vi "ULx-AIARG-UWKWT-Calibrate-Driver.vi"() -> ()   [LabVIEW 2017]
uses:
  <vilib>/Analysis/Matrix/Datatypes/RealMatrix.ctl
  <vilib>/Analysis/6fits.llb/Curve Fitting Criteria.ctl
  <vilib>/Analysis/baseanly.llb/Mean (DBL).vi
  <vilib>/ULx/Create Channel.llb/ULx Create Channel (AI-Voltage-Basic).vi
  <vilib>/ULx/Timing.llb/ULx Timing (Sample Clock).vi
  <vilib>/ULx/Read.llb/ULx Read (Analog Wfm 1Chan NSamp).vi
  <vilib>/Utility/file.llb/Write Delimited Spreadsheet (DBL).vi
  <vilib>/Analysis/Matrix/Numeric/Conversions/Array To Matrix - RA.vi
  <vilib>/Analysis/NI_AALBase.lvlib
  <vilib>/Analysis/Matrix/NI_Matrix.lvlib
  <vilib>/Analysis/NI_AALPro.lvlib
panel:
  out "CSV Array":dbl[][](array[numeric])
  in  "CSV Path":path
  in  "Rolling Moment Tab":T1(tab)
  out "Rolling Moment 1st Order Graph":T2(graph)
  out "Rolling Moment 1st Slope":dbl
  out "Rolling Moment 1st Intercept":dbl
  out "Rolling Moment 1st R-Squared":dbl
  out "Rolling Moment 2nd Order Graph":T2(graph)
  out "Rolling Moment 2nd Residue":dbl
  out "Rolling Moment 2nd Polynomial Coefficients":dbl[](array[numeric])
  out "Rolling Moment 3rd Order Graph":T2(graph)
  out "Rolling Moment 3rd Residue":dbl
  out "Rolling Moment 3rd Polynomial Coefficients":dbl[](array[numeric])
  in  "S.F. Tab":T3(tab)
  out "S.F. 1st Order Graph":cluster{"Weight":dbl[], "Voltage(S.F.)":dbl[]}[](graph)
  out "S.F. 1st Slope":dbl
  out "S.F. 1st Intercept":dbl
  out "S.F. 1st R-Squared":dbl
  out "S.F. 2nd Order Graph":cluster{"Weight":dbl[], "Voltage(S.F.)":dbl[]}[](graph)
  out "S.F. 2nd Polynomial Coefficients":dbl[](array[numeric])
  out "S.F. 2nd Residue":dbl
  out "S.F. 3rd Order Graph":cluster{"Weight":dbl[], "Voltage(S.F.)":dbl[]}[](graph)
  out "S.F. 3rd Polynomial Coefficients":dbl[](array[numeric])
  out "S.F. 3rd Residue":dbl
  in  "P.M. Tab":T4(tab)
  out "P.M. 1st Order Graph":cluster{"Weight":dbl[], "Voltage(P.M.)":dbl[]}[](graph)
  out "P.M. 1st Slope":dbl
  out "P.M. 1st Intercept":dbl
  out "P.M. 1st R-Squared":dbl
  out "P.M. 2nd Order Graph":cluster{"Weight":dbl[], "Voltage(P.M.)":dbl[]}[](graph)
  out "P.M. 2nd Polynomial Coefficients":dbl[](array[numeric])
  out "P.M. 2nd Residue":dbl
  out "P.M. 3rd Order Graph":cluster{"Weight":dbl[], "Voltage(P.M.)":dbl[]}[](graph)
  out "P.M. 3rd Polynomial Coefficients":dbl[](array[numeric])
  out "P.M. 3rd Residue":dbl
  in  "n Tab":enum32{"n Linear", "n 2nd Poly", "n 3rd Poly"}(tab)
  out "n 1st Order Graph":T5(graph)
  out "n 1st Slope":dbl
  out "n 1st Intercept":dbl
  out "n 1st R-Squared":dbl
  out "n 2nd Order Graph":T5(graph)
  out "n 2nd Residue":dbl
  out "n 2nd Polynomial Coefficients":dbl[](array[numeric])
  out "n 3rd Order Graph":T5(graph)
  out "n 3rd Polynomial Coefficients":dbl[](array[numeric])
  out "n 3rd Residue":dbl
  in  "Axial Tab":T6(tab)
  out "Axial 1st Order Graph":T7(graph)
  out "Axial 1st Slope":dbl
  out "Axial 1st Intercept":dbl
  out "Axial 1st R-Squared":dbl
  out "Axial 2nd Order Graph":T7(graph)
  out "Axial 2nd Residue":dbl
  out "Axial 2nd Polynomial Coefficients":dbl[](array[numeric])
  out "Axial 3rd Order Graph":T7(graph)
  out "Axial 3rd Polynomial Coefficients":dbl[](array[numeric])
  out "Axial 3rd Residue":dbl
  in  "Normal":T8(tab)
  out "Normal 1st Order Graph":T5(graph)
  out "Normal 1st Slope":dbl
  out "Normal 1st Intercept":dbl
  out "Normal 1st R-Squared":dbl
  out "Normal 2nd Order Graph":T5(graph)
  out "Normal 2nd Polynomial Coefficients":dbl[](array[numeric])
  out "Normal 2nd Residue":dbl
  out "Normal 3rd Order Graph":T5(graph)
  out "Normal 3rd Residue":dbl
  out "Normal 3rd Polynomial Coefficients":dbl[](array[numeric])
  out "Main Graph Intercept":dbl
  out "Main Graph R-Squared":dbl
  out "Main Graph Slope":dbl
  out "Main Graph":cluster{"Weight":dbl[], "Main Voltage":dbl[]}[](graph)
  out "Matrix Path Indicator":path
  in  "Report Path":path
  in  "Final Matrix":T9
  out "R.M. Sample Waveform":dbl[](graph)
  out "S.F. Sample Waveform":dbl[](graph)
  out "P.M. Sample Waveform":dbl[](graph)
  out "n Sample Waveform":dbl[](graph)
  out "Axial Force Sample Waveform":dbl[](graph)
  out "Normal Force Sample Waveform":dbl[](graph)
  out "Main Voltage":dbl[](array[numeric])
  out "Current Main Channel Calibration":string
  in  "Main Channel":string(combo)
  in  "Rolling Moment Physical Channel":refnum<k21>
  in  "S.F. Physical Channel":refnum<k21>
  in  "P.M. Physical Channel":refnum<k21>
  in  "n Physical Channel":refnum<k21>
  in  "Normal Force Physical Channel":refnum<k21>
  in  "minimum value":dbl=-5.0
  in  "maximum value":dbl=5.0
  in  "samples per channel":i32=100
  in  "sample mode":i32(ring) items=["FiniteSamples", "ContinuousSamples"]
  in  "rate":dbl=5000.0
  in  "Axial Force Physical Channel":refnum<k21>
  out "Voltage(R.M.)":dbl[](array[numeric])
  out "Voltage(S.F.)":dbl[](array[numeric])
  out "Voltage(P.M.)":dbl[](array[numeric])
  out "Voltage(n)":dbl[](array[numeric])
  out "Voltage(Normal)":dbl[](array[numeric])
  in  "Sample Button":bool
  in  "Add Weight":bool
  in  "Weight to be added":dbl
  out "Voltage(Axial)":dbl[](array[numeric])
  out "Weight":dbl[](array[numeric])
  in  "Clear Table":bool
  # "Channel and Sampling Selection"
  # "Interaction Plots\n\nPlots ALL SIX voltages,"
  # "Voltages from EACH Channel\nRecords data from all six channels for each sample cycle. Each number represents the mean of all values from one sample cycle recorded by one channel."
  # "Sample Waveform Graphs （For Debugging)\n\nPlots all the data points onto a waveform graph in one sample Cycle, to see the range of noises and determine any bias in data."
  # "Final Matrix\nThe final matrix that records the data from calibration and overwrites itself every time one calibration cycle is performed."
  # "Weight"
  # "Normal Force"
  # "Axial Force"
  # "n"
  # "P.M."
  # "S.F."
  # "Rolling Moment"
  # "f(x) ="
  # "*x +"
  # "f(x) ="
  # "*x +"
  # "f(x) ="
  # "*x +"
  # "f(x) ="
  # "*x +"
  # "f(x) ="
  # "*x +"
  # "f(x) ="
  # "*x +"
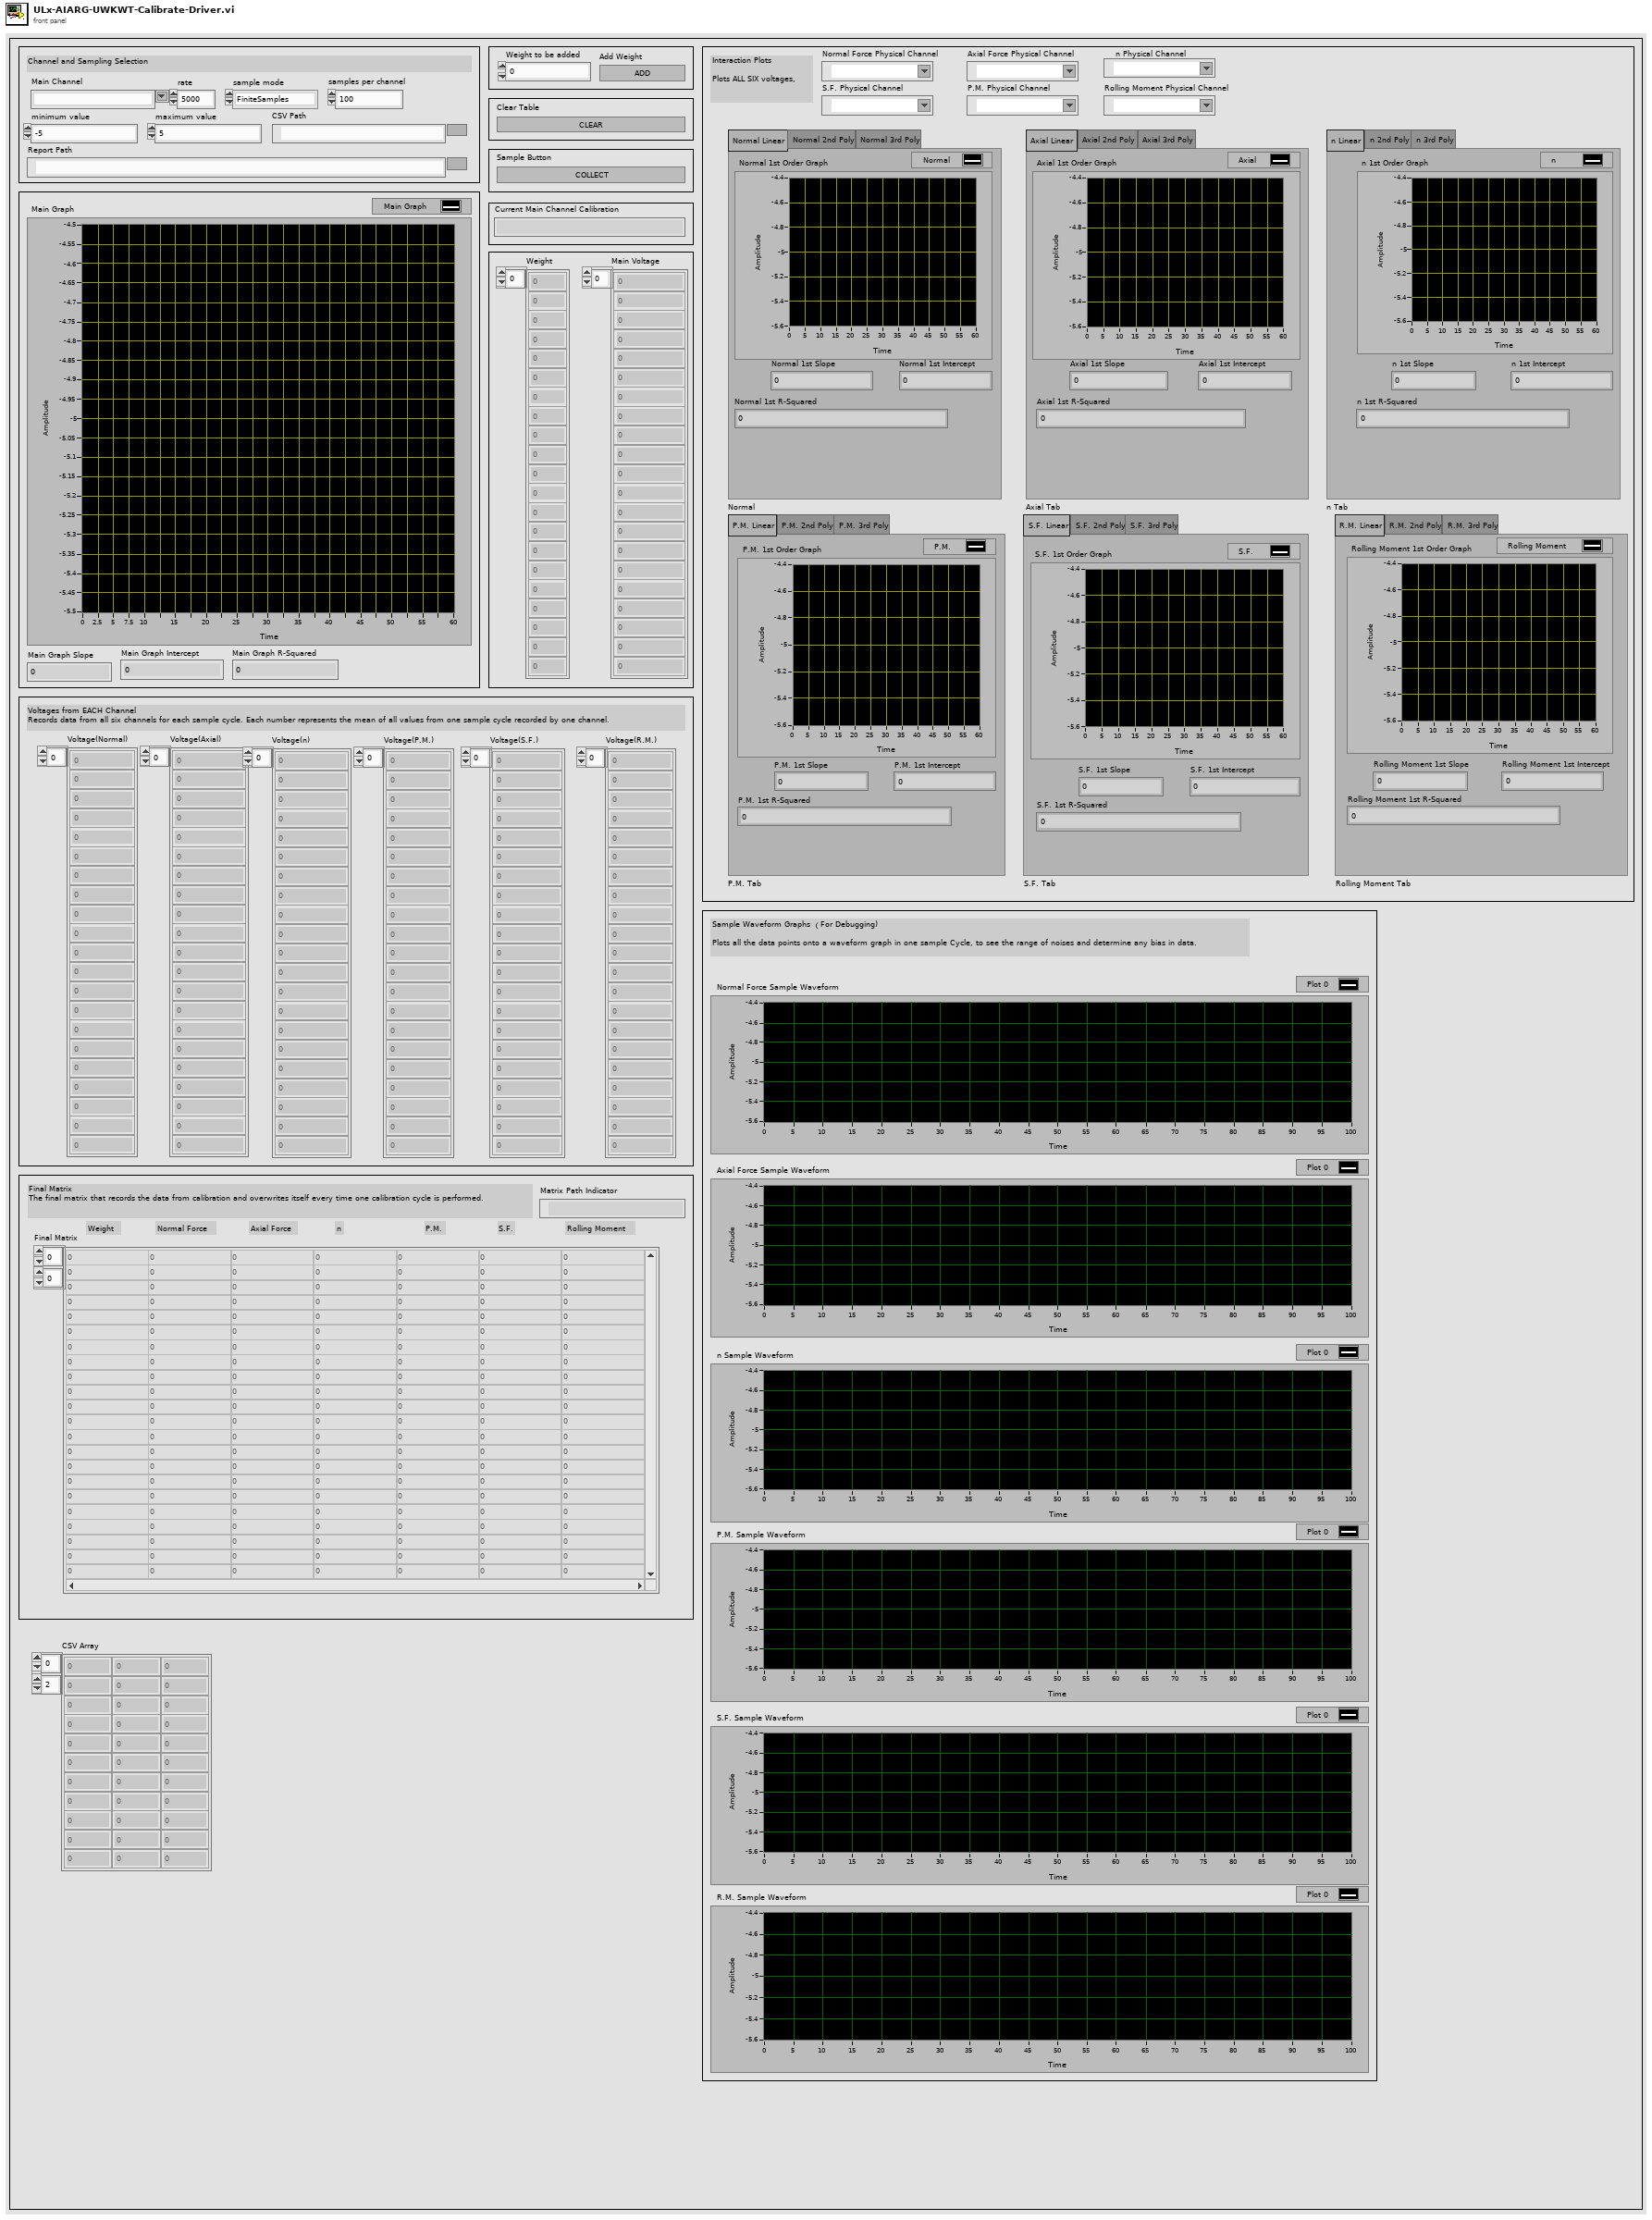
[diagram p1: front panel]
types:
  T1 = enum32{"R.M. Linear", "R.M. 2nd Poly", "R.M. 3rd Poly"}
  T2 = cluster{"Weight":dbl[], "Voltage(R.M.) ":dbl[]}[]
  T3 = enum32{"S.F. Linear", "S.F. 2nd Poly", "S.F. 3rd Poly"}
  T4 = enum32{"P.M. Linear", "P.M. 2nd Poly", "P.M. 3rd Poly"}
  T5 = cluster{"Weight":dbl[], "Best Linear Fit":dbl[]}[]
  T6 = enum32{"Axial Linear", "Axial 2nd Poly", "Axial 3rd Poly"}
  T7 = cluster{"Weight":dbl[], "Voltage(Axial)":dbl[]}[]
  T8 = enum32{"Normal Linear", "Normal 2nd Poly", "Normal 3rd Poly"}
  T9 = typedef "NI_Matrix.lvlib/RealMatrix.ctl" = dbl[][]
  T10 = typedef "NI_AALPro.lvlib/Curve Fitting Criteria.ctl" = u16
  T11 = cluster{"Weight":dbl[], "Best Polynomial Fit":dbl[]}
  T12 = cluster{"Weight":dbl[], "Best Polynomial Fit":dbl[]}[]
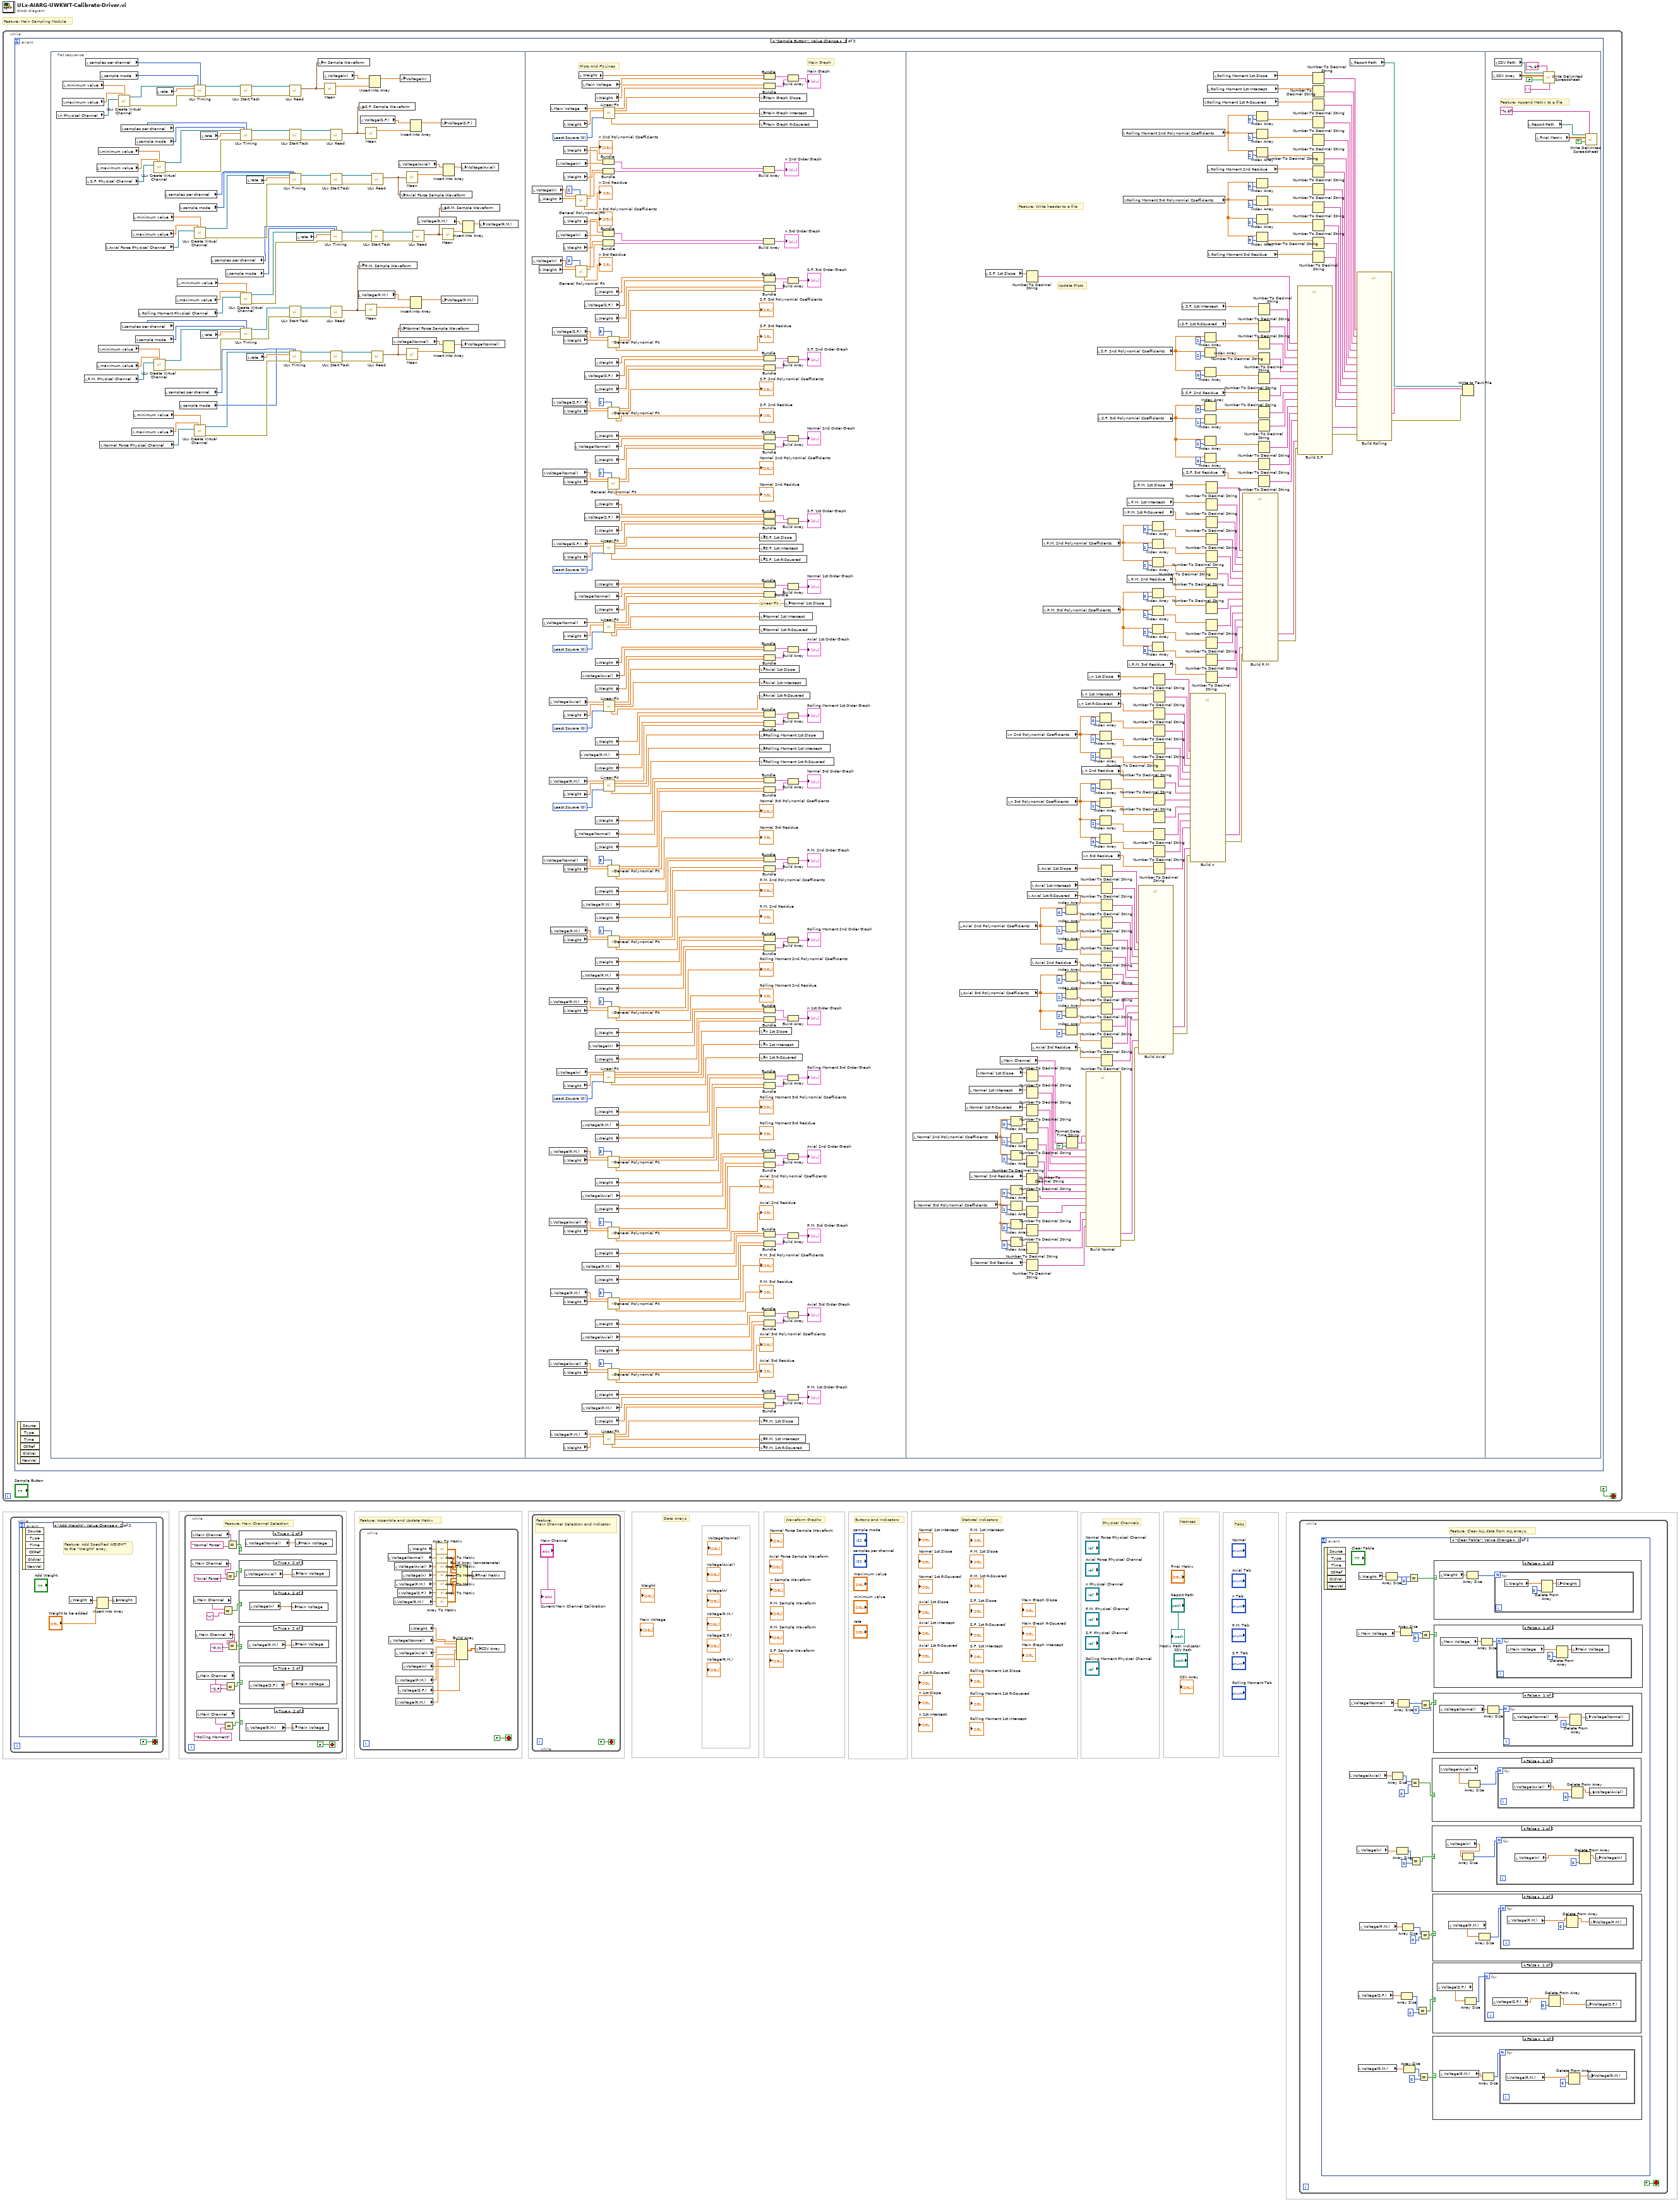
[diagram p0: block diagram]
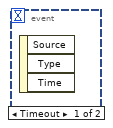
[diagram p8: hidden frame]
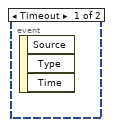
[diagram p17: hidden frame]
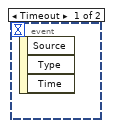
[diagram p18: hidden frame]
diagram:
  # "Tabs"
  # "Statistal Indicators"
  # "Matrices"
  # "Feature: Assemble and Update Matrix"
  # "Waveform Graphs"
  # "Physical Channels"
  # "Feature: Main Sampling Module"
  # "Data Arrays"
  # "Buttons and Indicators"
  n1 = while {
    stop <- FALSE stop-if-true
    n2 = event shown="[1] \"Sample Button\": Value Change" {
      selector: _ -> [_ _]
      dyn-events: _ -> [_ _]
      timeout: _ -> [_ _]
      event Timeout {
        n3 = event-data() -> ()  [unwired: 1 in, 3 out]
      }
      event "Sample Button": Value Change {
        n4 = event-data() -> ()  [unwired: 1 in, 6 out]
        n5 = flat-sequence {
          frame #0 {
            n6 = local read "n Physical Channel"() -> (w68:refnum<k21>)
            n7 = local read "maximum value"() -> (w64:dbl)
            n8 = local read "minimum value"() -> (w63:dbl)
            n9 = local read "P.M. Physical Channel"() -> (w53:refnum<k21>)
            n10 = local read "samples per channel"() -> (w66:i32)
            n11 = local read "S.F. Physical Channel"() -> (w28:refnum<k21>)
            n12 = local read "maximum value"() -> (w25:dbl)
            n13 = local read "maximum value"() -> (w52:dbl)
            n14 = local read "minimum value"() -> (w26:dbl)
            n15 = local read "minimum value"() -> (w51:dbl)
            n16 = local read "Normal Force Physical Channel"() -> (w83:refnum<k21>)
            n17 = local read "sample mode"() -> (w65:i32)
            n18 = local read "Axial Force Physical Channel"() -> (w84:refnum<k21>)
            n19 = call-poly <vilib>:"ULx Create Virtual Channel.vi"("maximum value"=w64, "minimum value"=w63, "physical channels"=w68) -> ("task out"=w54:refnum<k24>, "error out"=w55:errorcluster)  [unwired: 11 in]
            n20 = local read "samples per channel"() -> (w22:i32)
            n21 = local read "samples per channel"() -> (w43:i32)
            n22 = local read "maximum value"() -> (w88:dbl)
            n23 = local read "maximum value"() -> (w81:dbl)
            n24 = local read "minimum value"() -> (w95:dbl)
            n25 = local read "minimum value"() -> (w82:dbl)
            n26 = local read "sample mode"() -> (w21:i32)
            n27 = local read "sample mode"() -> (w42:i32)
            n28 = local read "Rolling Moment Physical Channel"() -> (w27:refnum<k21>)
            n29 = call-poly <vilib>:"ULx Create Virtual Channel.vi"("maximum value"=w25, "minimum value"=w26, "physical channels"=w28) -> ("task out"=w24:refnum<k24>, "error out"=w23:errorcluster)  [unwired: 11 in]
            n30 = call-poly <vilib>:"ULx Create Virtual Channel.vi"("maximum value"=w52, "minimum value"=w51, "physical channels"=w53) -> ("task out"=w50:refnum<k24>, "error out"=w41:errorcluster)  [unwired: 11 in]
            n31 = local read "rate"() -> (w67:dbl)
            n32 = local read "samples per channel"() -> (w85:i32)
            n33 = local read "samples per channel"() -> (w77:i32)
            n34 = local read "maximum value"() -> (w13:dbl)
            n35 = local read "minimum value"() -> (w14:dbl)
            n36 = local read "sample mode"() -> (w86:i32)
            n37 = local read "sample mode"() -> (w78:i32)
            n38 = call-poly <vilib>:"ULx Timing.vi"("task in"=w54, "sample mode"=w65, "samples per channel"=w66, "rate"=w67, "error in"=w55) -> ("task out"=w57:refnum<k24>, "error out"=w56:errorcluster)  [unwired: 9 in]
            n39 = call-poly <vilib>:"ULx Create Virtual Channel.vi"("maximum value"=w88, "minimum value"=w95, "physical channels"=w84) -> ("task out"=w89:refnum<k24>, "error out"=w94:errorcluster)  [unwired: 11 in]
            n40 = call-poly <vilib>:"ULx Create Virtual Channel.vi"("maximum value"=w81, "minimum value"=w82, "physical channels"=w83) -> ("task out"=w76:refnum<k24>, "error out"=w80:errorcluster)  [unwired: 11 in]
            n41 = local read "rate"() -> (w48:dbl)
            n42 = local read "rate"() -> (w49:dbl)
            n43 = local read "samples per channel"() -> (w16:i32)
            n44 = local read "sample mode"() -> (w15:i32)
            n45 = call <vilib>:"ULx Start Task.vi"("task in"=w57, "error in"=w56) -> ("task out"=w59:refnum<k24>, "error out"=w58:errorcluster)  [unwired: 12 in]
            n46 = call-poly <vilib>:"ULx Timing.vi"("task in"=w24, "sample mode"=w21, "samples per channel"=w22, "rate"=w48, "error in"=w23) -> ("task out"=w20:refnum<k24>, "error out"=w19:errorcluster)  [unwired: 9 in]
            n47 = call-poly <vilib>:"ULx Create Virtual Channel.vi"("maximum value"=w13, "minimum value"=w14, "physical channels"=w27) -> ("task out"=w12:refnum<k24>, "error out"=w11:errorcluster)  [unwired: 11 in]
            n48 = call-poly <vilib>:"ULx Timing.vi"("task in"=w50, "sample mode"=w42, "samples per channel"=w43, "rate"=w49, "error in"=w41) -> ("task out"=w40:refnum<k24>, "error out"=w39:errorcluster)  [unwired: 9 in]
            n49 = local read "rate"() -> (w87:dbl)
            n50 = local read "rate"() -> (w79:dbl)
            n51 = call-poly <vilib>:"ULx Read.vi"("task in"=w59, "error in"=w58) -> ("data"=w6:waveform(dbl))  [unwired: 11 in, 2 out]
            n52 = call <vilib>:"ULx Start Task.vi"("task in"=w20, "error in"=w19) -> ("task out"=w18:refnum<k24>, "error out"=w17:errorcluster)  [unwired: 12 in]
            n53 = call-poly <vilib>:"ULx Timing.vi"("task in"=w89, "sample mode"=w86, "samples per channel"=w85, "rate"=w87, "error in"=w94) -> ("task out"=w90:refnum<k24>, "error out"=w93:errorcluster)  [unwired: 9 in]
            n54 = call <vilib>:"ULx Start Task.vi"("task in"=w40, "error in"=w39) -> ("task out"=w38:refnum<k24>, "error out"=w37:errorcluster)  [unwired: 12 in]
            n55 = call-poly <vilib>:"ULx Timing.vi"("task in"=w76, "sample mode"=w78, "samples per channel"=w77, "rate"=w79, "error in"=w80) -> ("task out"=w75:refnum<k24>, "error out"=w74:errorcluster)  [unwired: 9 in]
            n56 = local read "rate"() -> (w47:dbl)
            n57 = local write "n Sample Waveform"(w6) -> ()
            n58 = local read "Voltage(n)"() -> (w62:dbl[])
            n59 = call-poly <vilib>:"Mean.vi"("X"=w6) -> ("mean"=w60:dbl)  [unwired: 1 out]
            n60 = call-poly <vilib>:"ULx Read.vi"("task in"=w18, "error in"=w17) -> ("data"=w3:waveform(dbl))  [unwired: 11 in, 2 out]
            n61 = call <vilib>:"ULx Start Task.vi"("task in"=w90, "error in"=w93) -> ("task out"=w91:refnum<k24>, "error out"=w92:errorcluster)  [unwired: 12 in]
            n62 = call-poly <vilib>:"ULx Timing.vi"("task in"=w12, "sample mode"=w15, "samples per channel"=w16, "rate"=w47, "error in"=w11) -> ("task out"=w10:refnum<k24>, "error out"=w9:errorcluster)  [unwired: 9 in]
            n63 = call-poly <vilib>:"ULx Read.vi"("task in"=w38, "error in"=w37) -> ("data"=w4:waveform(dbl))  [unwired: 11 in, 2 out]
            n64 = call <vilib>:"ULx Start Task.vi"("task in"=w75, "error in"=w74) -> ("task out"=w73:refnum<k24>, "error out"=w72:errorcluster)  [unwired: 12 in]
            n65 = local read "Voltage(P.M.)"() -> (w45:dbl[])
            n66 = local write "S.F. Sample Waveform"(w3) -> ()
            n67 = local write "P.M. Sample Waveform"(w4) -> ()
            n68 = local read "Voltage(S.F.)"() -> (w30:dbl[])
            n69 = call-poly <vilib>:"Mean.vi"("X"=w3) -> ("mean"=w31:dbl)  [unwired: 1 out]
            n70 = call-poly <vilib>:"Mean.vi"("X"=w4) -> ("mean"=w46:dbl)  [unwired: 1 out]
            n71 = Insert Into Array(array=w62, new element=w60) -> (w61:dbl[])  [unwired: 1 in]
            n72 = call-poly <vilib>:"ULx Read.vi"("task in"=w91, "error in"=w92) -> ("data"=w7:waveform(dbl))  [unwired: 11 in, 2 out]
            n73 = call <vilib>:"ULx Start Task.vi"("task in"=w10, "error in"=w9) -> ("task out"=w33:refnum<k24>, "error out"=w32:errorcluster)  [unwired: 12 in]
            n74 = call-poly <vilib>:"ULx Read.vi"("task in"=w73, "error in"=w72) -> ("data"=w8:waveform(dbl))  [unwired: 11 in, 2 out]
            n75 = local read "Voltage(Normal)"() -> (w70:dbl[])
            n76 = local read "Voltage(Axial)"() -> (w97:dbl[])
            n77 = local write "Voltage(n)"(w61) -> ()
            n78 = local write "Axial Force Sample Waveform"(w7) -> ()
            n79 = local write "Normal Force Sample Waveform"(w8) -> ()
            n80 = call-poly <vilib>:"Mean.vi"("X"=w7) -> ("mean"=w96:dbl)  [unwired: 1 out]
            n81 = call-poly <vilib>:"Mean.vi"("X"=w8) -> ("mean"=w71:dbl)  [unwired: 1 out]
            n82 = Insert Into Array(array=w30, new element=w31) -> (w29:dbl[])  [unwired: 1 in]
            n83 = Insert Into Array(array=w45, new element=w46) -> (w44:dbl[])  [unwired: 1 in]
            n84 = call-poly <vilib>:"ULx Read.vi"("task in"=w33, "error in"=w32) -> ("data"=w5:waveform(dbl))  [unwired: 11 in, 2 out]
            n85 = local read "Voltage(R.M.)"() -> (w35:dbl[])
            n86 = local write "Voltage(S.F.)"(w29) -> ()
            n87 = local write "R.M. Sample Waveform"(w5) -> ()
            n88 = local write "Voltage(P.M.)"(w44) -> ()
            n89 = call-poly <vilib>:"Mean.vi"("X"=w5) -> ("mean"=w34:dbl)  [unwired: 1 out]
            n90 = Insert Into Array(array=w97, new element=w96) -> (w98:dbl[])  [unwired: 1 in]
            n91 = Insert Into Array(array=w70, new element=w71) -> (w69:dbl[])  [unwired: 1 in]
            n92 = local write "Voltage(Axial)"(w98) -> ()
            n93 = local write "Voltage(Normal)"(w69) -> ()
            n94 = Insert Into Array(array=w35, new element=w34) -> (w36:dbl[])  [unwired: 1 in]
            n95 = local write "Voltage(R.M.)"(w36) -> ()
          }
          frame #1 {
            w223 = T10 0 items=["Least Square", "Least Absolute Residual", "Bisquare"] ("method")
            w247 = T10 0 items=["Least Square", "Least Absolute Residual", "Bisquare"] ("method")
            w275 = T10 0 items=["Least Square", "Least Absolute Residual", "Bisquare"] ("method")
            w286 = T10 0 items=["Least Square", "Least Absolute Residual", "Bisquare"] ("method")
            w297 = T10 0 items=["Least Square", "Least Absolute Residual", "Bisquare"] ("method")
            w312 = T10 0 items=["Least Square", "Least Absolute Residual", "Bisquare"] ("method")
            # "Main Graph"
            # "Linear Fit"
            # "Plots And Fit Lines"
            n96 = local read "Voltage(n)"() -> (w214:dbl[])
            n97 = local read "Voltage(n)"() -> (w139:dbl[])
            n98 = local read "Weight"() -> (w213:dbl[])
            n99 = local read "Weight"() -> (w138:dbl[])
            n100 = local read "Voltage(Normal)"() -> (w236:dbl[])
            n101 = local read "Voltage(Normal)"() -> (w301:dbl[])
            n102 = local read "Voltage(Normal)"() -> (w160:dbl[])
            n103 = local read "Voltage(Axial)"() -> (w288:dbl[])
            n104 = local read "Voltage(R.M.)"() -> (w246:dbl[])
            n105 = local read "Voltage(R.M.)"() -> (w179:dbl[])
            n106 = local read "Voltage(R.M.)"() -> (w106:dbl[])
            n107 = local read "Voltage(Axial)"() -> (w207:dbl[])
            n108 = local read "Voltage(Axial)"() -> (w150:dbl[])
            n109 = local read "Main Voltage"() -> (w316:dbl[])
            n110 = local read "Voltage(P.M.)"() -> (w186:dbl[])
            n111 = local read "Voltage(P.M.)"() -> (w127:dbl[])
            n112 = local read "Voltage(P.M.)"() -> (w266:dbl[])
            n113 = local read "Voltage(S.F.)"() -> (w113:dbl[])
            n114 = local read "Voltage(S.F.)"() -> (w201:dbl[])
            n115 = local read "Voltage(S.F.)"() -> (w259:dbl[])
            n116 = local read "Voltage(n)"() -> (w218:dbl[])
            n117 = local read "Voltage(n)"() -> (w144:dbl[])
            n118 = local read "Voltage(n)"() -> (w279:dbl[])
            n119 = local read "Weight"() -> (w317:dbl[])
            n120 = local read "Weight"() -> (w220:dbl[])
            n121 = local read "Weight"() -> (w215:dbl[])
            n122 = local read "Weight"() -> (w145:dbl[])
            n123 = local read "Weight"() -> (w143:dbl[])
            n124 = local read "Weight"() -> (w114:dbl[])
            n125 = local read "Weight"() -> (w200:dbl[])
            n126 = local read "Weight"() -> (w235:dbl[])
            n127 = local read "Weight"() -> (w258:dbl[])
            n128 = local read "Weight"() -> (w302:dbl[])
            n129 = local read "Weight"() -> (w287:dbl[])
            n130 = local read "Weight"() -> (w248:dbl[])
            n131 = local read "Weight"() -> (w159:dbl[])
            n132 = local read "Weight"() -> (w185:dbl[])
            n133 = local read "Weight"() -> (w178:dbl[])
            n134 = local read "Weight"() -> (w280:dbl[])
            n135 = local read "Weight"() -> (w107:dbl[])
            n136 = local read "Weight"() -> (w225:dbl[])
            n137 = local read "Weight"() -> (w126:dbl[])
            n138 = local read "Weight"() -> (w149:dbl[])
            n139 = local read "Weight"() -> (w265:dbl[])
            n140 = local read "Voltage(Normal)"() -> (w242:dbl[])
            n141 = local read "Voltage(Normal)"() -> (w330:dbl[])
            n142 = local read "Voltage(Normal)"() -> (w169:dbl[])
            n143 = call <vilib>:"General Polynomial Fit.vi"("Y"=w214, "polynomial order"=2, "X"=w213) -> ("Best Polynomial Fit"=w216:dbl[], "Polynomial Coefficients"=→"n 2nd Polynomial Coefficients":dbl[], "residue"=→"n 2nd Residue":dbl)  [unwired: 9 in, 1 out]
            n144 = call <vilib>:"General Polynomial Fit.vi"("Y"=w139, "polynomial order"=3, "X"=w138) -> ("Best Polynomial Fit"=w141:dbl[], "Polynomial Coefficients"=→"n 3rd Polynomial Coefficients":dbl[], "residue"=→"n 3rd Residue":dbl)  [unwired: 9 in, 1 out]
            n145 = local read "Weight"() -> (w311:dbl[])
            n146 = local read "Voltage(R.M.)"() -> (w320:dbl[])
            n147 = local read "Voltage(Axial)"() -> (w328:dbl[])
            n148 = local read "Voltage(R.M.)"() -> (w181:dbl[])
            n149 = local read "Voltage(R.M.)"() -> (w109:dbl[])
            n150 = local read "Voltage(Axial)"() -> (w208:dbl[])
            n151 = local read "Voltage(Axial)"() -> (w157:dbl[])
            n152 = local read "Main Voltage"() -> (w332:dbl[])
            n153 = local read "Voltage(P.M.)"() -> (w190:dbl[])
            n154 = local read "Voltage(P.M.)"() -> (w133:dbl[])
            n155 = local read "Voltage(P.M.)"() -> (w324:dbl[])
            n156 = local read "Voltage(S.F.)"() -> (w121:dbl[])
            n157 = local read "Voltage(S.F.)"() -> (w205:dbl[])
            n158 = local read "Voltage(S.F.)"() -> (w322:dbl[])
            n159 = local read "Voltage(n)"() -> (w326:dbl[])
            n160 = local read "Weight"() -> (w309:dbl[])
            n161 = local read "Weight"() -> (w122:dbl[])
            n162 = local read "Weight"() -> (w119:dbl[])
            n163 = local read "Weight"() -> (w206:dbl[])
            n164 = local read "Weight"() -> (w203:dbl[])
            n165 = local read "Weight"() -> (w243:dbl[])
            n166 = local read "Weight"() -> (w239:dbl[])
            n167 = local read "Weight"() -> (w323:dbl[])
            n168 = local read "Weight"() -> (w260:dbl[])
            n169 = local read "Weight"() -> (w331:dbl[])
            n170 = local read "Weight"() -> (w307:dbl[])
            n171 = local read "Weight"() -> (w329:dbl[])
            n172 = local read "Weight"() -> (w293:dbl[])
            n173 = local read "Weight"() -> (w321:dbl[])
            n174 = local read "Weight"() -> (w245:dbl[])
            n175 = local read "Weight"() -> (w170:dbl[])
            n176 = local read "Weight"() -> (w168:dbl[])
            n177 = local read "Weight"() -> (w191:dbl[])
            n178 = local read "Weight"() -> (w189:dbl[])
            n179 = local read "Weight"() -> (w182:dbl[])
            n180 = local read "Weight"() -> (w177:dbl[])
            n181 = local read "Weight"() -> (w327:dbl[])
            n182 = local read "Weight"() -> (w285:dbl[])
            n183 = local read "Weight"() -> (w110:dbl[])
            n184 = local read "Weight"() -> (w108:dbl[])
            n185 = local read "Weight"() -> (w231:dbl[])
            n186 = local read "Weight"() -> (w230:dbl[])
            n187 = local read "Weight"() -> (w134:dbl[])
            n188 = local read "Weight"() -> (w131:dbl[])
            n189 = local read "Weight"() -> (w158:dbl[])
            n190 = local read "Weight"() -> (w156:dbl[])
            n191 = local read "Weight"() -> (w325:dbl[])
            n192 = local read "Weight"() -> (w271:dbl[])
            n193 = Bundle("Weight"=w220, "Voltage(n)"=w218) -> (w219:cluster{"Weight":dbl[], "Voltage(n)":dbl[]})  [unwired: 1 in]
            n194 = Bundle("Weight"=w215, "Best Polynomial Fit"=w216) -> (w217:T11)  [unwired: 1 in]
            n195 = Bundle("Weight"=w145, "Voltage(n)"=w144) -> (w146:cluster{"Weight":dbl[], "Voltage(n)":dbl[]})  [unwired: 1 in]
            n196 = Bundle("Weight"=w143, "Best Polynomial Fit"=w141) -> (w142:T11)  [unwired: 1 in]
            n197 = call <vilib>:"Linear Fit.vi"("Y"=w316, "X"=w317, "method"=w312) -> ("Best Linear Fit"=w308:dbl[], "slope"=w315:dbl, "intercept"=w314:dbl, "residue"=w313:dbl)  [unwired: 8 in, 1 out]
            n198 = call <vilib>:"Linear Fit.vi"("Y"=w259, "X"=w258, "method"=w247) -> ("Best Linear Fit"=w261:dbl[], "slope"=w257:dbl, "intercept"=w256:dbl, "residue"=w255:dbl)  [unwired: 8 in, 1 out]
            n199 = call <vilib>:"Linear Fit.vi"("Y"=w301, "X"=w302, "method"=w297) -> ("Best Linear Fit"=w304:dbl[], "slope"=w303:dbl, "intercept"=w305:dbl, "residue"=w306:dbl)  [unwired: 8 in, 1 out]
            n200 = call <vilib>:"Linear Fit.vi"("Y"=w288, "X"=w287, "method"=w286) -> ("Best Linear Fit"=w292:dbl[], "slope"=w291:dbl, "intercept"=w290:dbl, "residue"=w289:dbl)  [unwired: 8 in, 1 out]
            n201 = call <vilib>:"Linear Fit.vi"("Y"=w246, "X"=w248, "method"=w223) -> ("Best Linear Fit"=w252:dbl[], "slope"=w251:dbl, "intercept"=w250:dbl, "residue"=w249:dbl)  [unwired: 8 in, 1 out]
            n202 = call <vilib>:"Linear Fit.vi"("Y"=w279, "X"=w280, "method"=w275) -> ("Best Linear Fit"=w284:dbl[], "slope"=w283:dbl, "intercept"=w282:dbl, "residue"=w281:dbl)  [unwired: 8 in, 1 out]
            n203 = call <vilib>:"Linear Fit.vi"("Y"=w266, "X"=w265) -> ("Best Linear Fit"=w272:dbl[], "slope"=w269:dbl, "intercept"=w268:dbl, "residue"=w267:dbl)  [unwired: 9 in, 1 out]
            n204 = call <vilib>:"General Polynomial Fit.vi"("Y"=w113, "polynomial order"=3, "X"=w114) -> ("Best Polynomial Fit"=w118:dbl[], "Polynomial Coefficients"=→"S.F. 3rd Polynomial Coefficients":dbl[], "residue"=→"S.F. 3rd Residue":dbl)  [unwired: 9 in, 1 out]
            n205 = call <vilib>:"General Polynomial Fit.vi"("Y"=w201, "polynomial order"=2, "X"=w200) -> ("Best Polynomial Fit"=w202:dbl[], "Polynomial Coefficients"=→"S.F. 2nd Polynomial Coefficients":dbl[], "residue"=→"S.F. 2nd Residue":dbl)  [unwired: 9 in, 1 out]
            n206 = call <vilib>:"General Polynomial Fit.vi"("Y"=w236, "polynomial order"=2, "X"=w235) -> ("Best Polynomial Fit"=w238:dbl[], "Polynomial Coefficients"=→"Normal 2nd Polynomial Coefficients":dbl[], "residue"=→"Normal 2nd Residue":dbl)  [unwired: 9 in, 1 out]
            n207 = call <vilib>:"General Polynomial Fit.vi"("Y"=w160, "polynomial order"=3, "X"=w159) -> ("Best Polynomial Fit"=w167:dbl[], "Polynomial Coefficients"=→"Normal 3rd Polynomial Coefficients":dbl[], "residue"=→"Normal 3rd Residue":dbl)  [unwired: 9 in, 1 out]
            n208 = call <vilib>:"General Polynomial Fit.vi"("Y"=w186, "polynomial order"=2, "X"=w185) -> ("Best Polynomial Fit"=w188:dbl[], "Polynomial Coefficients"=→"P.M. 2nd Polynomial Coefficients":dbl[], "residue"=→"P.M. 2nd Residue":dbl)  [unwired: 9 in, 1 out]
            n209 = call <vilib>:"General Polynomial Fit.vi"("Y"=w179, "polynomial order"=2, "X"=w178) -> ("Best Polynomial Fit"=w180:dbl[], "Polynomial Coefficients"=→"Rolling Moment 2nd Polynomial Coefficients":dbl[], "residue"=→"Rolling Moment 2nd Residue":dbl)  [unwired: 9 in, 1 out]
            n210 = call <vilib>:"General Polynomial Fit.vi"("Y"=w106, "polynomial order"=3, "X"=w107) -> ("Best Polynomial Fit"=w104:dbl[], "Polynomial Coefficients"=→"Rolling Moment 3rd Polynomial Coefficients":dbl[], "residue"=→"Rolling Moment 3rd Residue":dbl)  [unwired: 9 in, 1 out]
            n211 = call <vilib>:"General Polynomial Fit.vi"("Y"=w207, "polynomial order"=2, "X"=w225) -> ("Best Polynomial Fit"=w227:dbl[], "Polynomial Coefficients"=→"Axial 2nd Polynomial Coefficients":dbl[], "residue"=→"Axial 2nd Residue":dbl)  [unwired: 9 in, 1 out]
            n212 = call <vilib>:"General Polynomial Fit.vi"("Y"=w127, "polynomial order"=3, "X"=w126) -> ("Best Polynomial Fit"=w132:dbl[], "Polynomial Coefficients"=→"P.M. 3rd Polynomial Coefficients":dbl[], "residue"=→"P.M. 3rd Residue":dbl)  [unwired: 9 in, 1 out]
            n213 = call <vilib>:"General Polynomial Fit.vi"("Y"=w150, "polynomial order"=3, "X"=w149) -> ("Best Polynomial Fit"=w154:dbl[], "Polynomial Coefficients"=→"Axial 3rd Polynomial Coefficients":dbl[], "residue"=→"Axial 3rd Residue":dbl)  [unwired: 9 in, 1 out]
            n214 = local write "Main Graph Slope"(w315) -> ()
            n215 = local write "Main Graph Intercept"(w314) -> ()
            n216 = local write "Main Graph R-Squared"(w313) -> ()
            n217 = local write "S.F. 1st Slope"(w257) -> ()
            n218 = local write "S.F. 1st Intercept"(w256) -> ()
            n219 = local write "S.F. 1st R-Squared"(w255) -> ()
            n220 = local write "Normal 1st Intercept"(w305) -> ()
            n221 = local write "Normal 1st R-Squared"(w306) -> ()
            n222 = local write "Axial 1st Slope"(w291) -> ()
            n223 = local write "Axial 1st Intercept"(w290) -> ()
            n224 = local write "Axial 1st R-Squared"(w289) -> ()
            n225 = local write "Rolling Moment 1st Slope"(w251) -> ()
            n226 = local write "Rolling Moment 1st Intercept"(w250) -> ()
            n227 = local write "Rolling Moment 1st R-Squared"(w249) -> ()
            n228 = local write "n 1st Slope"(w283) -> ()
            n229 = local write "n 1st Intercept"(w282) -> ()
            n230 = local write "n 1st R-Squared"(w281) -> ()
            n231 = local write "P.M. 1st Slope"(w269) -> ()
            n232 = local write "P.M. 1st Intercept"(w268) -> ()
            n233 = local write "P.M. 1st R-Squared"(w267) -> ()
            n234 = Build Array(w219, w217) -> (→"n 2nd Order Graph":T12)
            n235 = Build Array(w146, w142) -> (→"n 3rd Order Graph":T12)
            n236 = Bundle("Weight"=w311, "Main Voltage"=w332) -> (w318:cluster{"Weight":dbl[], "Main Voltage":dbl[]})  [unwired: 1 in]
            n237 = Bundle("Weight"=w309, "Best Linear Fit"=w308) -> (w310:cluster{"Weight":dbl[], "Best Linear Fit":dbl[]})  [unwired: 1 in]
            n238 = Bundle("Weight"=w122, "Voltage(S.F.)"=w121) -> (w120:cluster{"Weight":dbl[], "Voltage(S.F.)":dbl[]})  [unwired: 1 in]
            n239 = Bundle("Weight"=w119, "Best Polynomial Fit"=w118) -> (w111:T11)  [unwired: 1 in]
            n240 = Bundle("Weight"=w206, "Voltage(S.F.)"=w205) -> (w204:cluster{"Weight":dbl[], "Voltage(S.F.)":dbl[]})  [unwired: 1 in]
            n241 = Bundle("Weight"=w203, "Best Polynomial Fit"=w202) -> (w199:T11)  [unwired: 1 in]
            n242 = Bundle("Weight"=w243, "Voltage(Normal)"=w242) -> (w241:cluster{"Weight":dbl[], "Voltage(Normal)":dbl[]})  [unwired: 1 in]
            n243 = Bundle("Weight"=w239, "Best Polynomial Fit"=w238) -> (w237:T11)  [unwired: 1 in]
            n244 = Bundle("Weight"=w323, "Voltage(S.F.)"=w322) -> (w263:cluster{"Weight":dbl[], "Voltage(S.F.)":dbl[]})  [unwired: 1 in]
            n245 = Bundle("Weight"=w260, "Best Linear Fit"=w261) -> (w262:cluster{"Weight":dbl[], "Best Linear Fit":dbl[]})  [unwired: 1 in]
            n246 = Bundle("Weight"=w331, "Voltage(Normal)"=w330) -> (w300:cluster{"Weight":dbl[], "Voltage(Normal)":dbl[]})  [unwired: 1 in]
            n247 = Bundle("Weight"=w307, "Best Linear Fit"=w304) -> (w299:cluster{"Weight":dbl[], "Best Linear Fit":dbl[]})  [unwired: 1 in]
            n248 = Bundle("Weight"=w329, "Voltage(Axial)"=w328) -> (w295:cluster{"Weight":dbl[], "Voltage(Axial)":dbl[]})  [unwired: 1 in]
            n249 = Bundle("Weight"=w293, "Best Linear Fit"=w292) -> (w294:cluster{"Weight":dbl[], "Best Linear Fit":dbl[]})  [unwired: 1 in]
            n250 = Bundle("Weight"=w321, "Voltage(R.M.)"=w320) -> (w253:cluster{"Weight":dbl[], "Voltage(R.M.) ":dbl[]})  [unwired: 1 in]
            n251 = Bundle("Weight"=w245, "Best Linear Fit"=w252) -> (w244:cluster{"Weight":dbl[], "Best Linear Fit":dbl[]})  [unwired: 1 in]
            n252 = Bundle("Weight"=w170, "Voltage(Normal)"=w169) -> (w163:cluster{"Weight":dbl[], "Voltage(Normal)":dbl[]})  [unwired: 1 in]
            n253 = Bundle("Weight"=w168, "Best Polynomial Fit"=w167) -> (w161:T11)  [unwired: 1 in]
            n254 = Bundle("Weight"=w191, "Voltage(P.M.)"=w190) -> (w193:cluster{"Weight":dbl[], "Voltage(P.M.)":dbl[]})  [unwired: 1 in]
            n255 = Bundle("Weight"=w189, "Best Polynomial Fit"=w188) -> (w192:T11)  [unwired: 1 in]
            n256 = Bundle("Weight"=w182, "Voltage(R.M.)"=w181) -> (w172:cluster{"Weight":dbl[], "Voltage(R.M.) ":dbl[]})  [unwired: 1 in]
            n257 = Bundle("Weight"=w177, "Best Polynomial Fit"=w180) -> (w173:T11)  [unwired: 1 in]
            n258 = Bundle("Weight"=w327, "Voltage(n)"=w326) -> (w278:cluster{"Weight":dbl[], "Voltage(n)":dbl[]})  [unwired: 1 in]
            n259 = Bundle("Weight"=w285, "Best Linear Fit"=w284) -> (w277:cluster{"Weight":dbl[], "Best Linear Fit":dbl[]})  [unwired: 1 in]
            n260 = Bundle("Weight"=w110, "Voltage(R.M.)"=w109) -> (w103:cluster{"Weight":dbl[], "Voltage(R.M.) ":dbl[]})  [unwired: 1 in]
            n261 = Bundle("Weight"=w108, "Best Polynomial Fit"=w104) -> (w102:T11)  [unwired: 1 in]
            n262 = Bundle("Weight"=w231, "Voltage(Axial)"=w208) -> (w229:cluster{"Weight":dbl[], "Voltage(Axial)":dbl[]})  [unwired: 1 in]
            n263 = Bundle("Weight"=w230, "Best Polynomial Fit"=w227) -> (w228:T11)  [unwired: 1 in]
            n264 = Bundle("Weight"=w134, "Voltage(P.M.)"=w133) -> (w130:cluster{"Weight":dbl[], "Voltage(P.M.)":dbl[]})  [unwired: 1 in]
            n265 = Bundle("Weight"=w131, "Best Polynomial Fit"=w132) -> (w129:T11)  [unwired: 1 in]
            n266 = Bundle("Weight"=w158, "Voltage(Axial)"=w157) -> (w153:cluster{"Weight":dbl[], "Voltage(Axial)":dbl[]})  [unwired: 1 in]
            n267 = Bundle("Weight"=w156, "Best Polynomial Fit"=w154) -> (w152:T11)  [unwired: 1 in]
            n268 = Bundle("Weight"=w325, "Voltage(P.M.)"=w324) -> (w273:cluster{"Weight":dbl[], "Voltage(P.M.)":dbl[]})  [unwired: 1 in]
            n269 = Bundle("Weight"=w271, "Best Linear Fit"=w272) -> (w270:cluster{"Weight":dbl[], "Best Linear Fit":dbl[]})  [unwired: 1 in]
            n270 = local write "Normal 1st Slope"(w303) -> ()
            n271 = Build Array(w318, w310) -> (→"Main Graph":T5)
            n272 = Build Array(w120, w111) -> (→"S.F. 3rd Order Graph":T12)
            n273 = Build Array(w204, w199) -> (→"S.F. 2nd Order Graph":T12)
            n274 = Build Array(w241, w237) -> (→"Normal 2nd Order Graph":T12)
            n275 = Build Array(w263, w262) -> (→"S.F. 1st Order Graph":T5)
            n276 = Build Array(w300, w299) -> (→"Normal 1st Order Graph":T5)
            n277 = Build Array(w295, w294) -> (→"Axial 1st Order Graph":T5)
            n278 = Build Array(w253, w244) -> (→"Rolling Moment 1st Order Graph":T5)
            n279 = Build Array(w163, w161) -> (→"Normal 3rd Order Graph":T12)
            n280 = Build Array(w193, w192) -> (→"P.M. 2nd Order Graph":T12)
            n281 = Build Array(w172, w173) -> (→"Rolling Moment 2nd Order Graph":T12)
            n282 = Build Array(w278, w277) -> (→"n 1st Order Graph":T5)
            n283 = Build Array(w103, w102) -> (→"Rolling Moment 3rd Order Graph":T12)
            n284 = Build Array(w229, w228) -> (→"Axial 2nd Order Graph":T12)
            n285 = Build Array(w130, w129) -> (→"P.M. 3rd Order Graph":T12)
            n286 = Build Array(w153, w152) -> (→"Axial 3rd Order Graph":T12)
            n287 = Build Array(w273, w270) -> (→"P.M. 1st Order Graph":T5)
          }
          frame #2 {
            # "Feature: Write header to a file"
            # "Update Plots"
            n288 = local read "Normal 2nd Polynomial Coefficients"() -> (w531:dbl[])
            n289 = local read "Normal 3rd Polynomial Coefficients"() -> (w523:dbl[])
            n290 = local read "Axial 2nd Polynomial Coefficients"() -> (w499:dbl[])
            n291 = local read "Axial 3rd Polynomial Coefficients"() -> (w489:dbl[])
            n292 = local read "Normal 1st R-Squared"() -> (w539:dbl)
            n293 = local read "Normal 1st Intercept"() -> (w541:dbl)
            n294 = local read "Normal 2nd Residue"() -> (w537:dbl)
            n295 = local read "Normal 3rd Residue"() -> (w534:dbl)
            n296 = local read "Normal 1st Slope"() -> (w543:dbl)
            n297 = local read "S.F. 1st Slope"() -> (w403:dbl)
            n298 = local read "Main Channel"() -> (w545:string)
            n299 = local read "n 2nd Polynomial Coefficients"() -> (w457:dbl[])
            n300 = local read "n 3rd Polynomial Coefficients"() -> (w450:dbl[])
            n301 = Index Array(array=w531, index=0) -> (element=w533:dbl)
            n302 = Index Array(array=w531, index=1) -> (element=w528:dbl)
            n303 = Index Array(array=w531, index=2) -> (element=w527:dbl)
            n304 = Index Array(array=w523, index=0) -> (element=w518:dbl)
            n305 = Index Array(array=w523, index=1) -> (element=w517:dbl)
            n306 = Index Array(array=w523, index=2) -> (element=w516:dbl)
            n307 = Index Array(array=w523, index=3) -> (element=w515:dbl)
            n308 = Number To Decimal String(number=w403) -> (decimal integer string=w400:string)  [unwired: 1 in]
            n309 = Number To Decimal String(number=w543) -> (decimal integer string=w542:string)  [unwired: 1 in]
            n310 = Number To Decimal String(number=w541) -> (decimal integer string=w540:string)  [unwired: 1 in]
            n311 = Number To Decimal String(number=w539) -> (decimal integer string=w538:string)  [unwired: 1 in]
            n312 = Number To Decimal String(number=w533) -> (decimal integer string=w526:string)  [unwired: 1 in]
            n313 = Number To Decimal String(number=w528) -> (decimal integer string=w525:string)  [unwired: 1 in]
            n314 = Number To Decimal String(number=w527) -> (decimal integer string=w524:string)  [unwired: 1 in]
            n315 = Number To Decimal String(number=w537) -> (decimal integer string=w536:string)  [unwired: 1 in]
            n316 = Number To Decimal String(number=w518) -> (decimal integer string=w514:string)  [unwired: 1 in]
            n317 = Number To Decimal String(number=w517) -> (decimal integer string=w513:string)  [unwired: 1 in]
            n318 = Number To Decimal String(number=w516) -> (decimal integer string=w512:string)  [unwired: 1 in]
            n319 = Number To Decimal String(number=w515) -> (decimal integer string=w511:string)  [unwired: 1 in]
            n320 = Number To Decimal String(number=w534) -> (decimal integer string=w535:string)  [unwired: 1 in]
            n321 = local read "Axial 1st R-Squared"() -> (w505:dbl)
            n322 = local read "Axial 1st Intercept"() -> (w507:dbl)
            n323 = local read "Axial 2nd Residue"() -> (w503:dbl)
            n324 = local read "Axial 3rd Residue"() -> (w501:dbl)
            n325 = local read "Axial 1st Slope"() -> (w509:dbl)
            n326 = local read "P.M. 2nd Polynomial Coefficients"() -> (w428:dbl[])
            n327 = local read "P.M. 3rd Polynomial Coefficients"() -> (w427:dbl[])
            n328 = Index Array(array=w499, index=0) -> (element=w495:dbl)
            n329 = Index Array(array=w499, index=1) -> (element=w494:dbl)
            n330 = Index Array(array=w499, index=2) -> (element=w493:dbl)
            n331 = Index Array(array=w489, index=0) -> (element=w484:dbl)
            n332 = Index Array(array=w489, index=1) -> (element=w483:dbl)
            n333 = Index Array(array=w489, index=2) -> (element=w482:dbl)
            n334 = Index Array(array=w489, index=3) -> (element=w481:dbl)
            n335 = Format Date/Time String(UTC format=TRUE) -> (date/time string=w544:string)  [unwired: 2 in]
            n336 = local read "n 1st R-Squared"() -> (w472:dbl)
            n337 = local read "n 1st Intercept"() -> (w473:dbl)
            n338 = local read "n 2nd Residue"() -> (w471:dbl)
            n339 = local read "n 3rd Residue"() -> (w470:dbl)
            n340 = call "Build Normal"("date"=w544, "mainchannel"=w545, "normal_1st_1st_coef"=w542, "normal_1st_2nd_coef"=w540, "normal_1st_residue"=w538, "normal_2nd_1st_coef"=w526, "normal_2nd_2nd_coef"=w525, "normal_2nd_3rd_coef"=w524, "normal_2nd_residue"=w536, "normal_3rd_1st_coef"=w514, "normal_3rd_2nd_coef"=w513, "normal_3rd_3rd_coef"=w512, "normal_3rd_4th_coef"=w511, "normal_3rd_residue"=w535) -> ("Result"=w510:string, "error out"=w476:errorcluster)  [unwired: 12 in]
            n341 = local read "n 1st Slope"() -> (w474:dbl)
            n342 = local read "S.F. 2nd Polynomial Coefficients"() -> (w387:dbl[])
            n343 = local read "S.F. 3rd Polynomial Coefficients"() -> (w378:dbl[])
            n344 = Index Array(array=w457, index=0) -> (element=w454:dbl)
            n345 = Index Array(array=w457, index=1) -> (element=w455:dbl)
            n346 = Index Array(array=w457, index=2) -> (element=w456:dbl)
            n347 = Index Array(array=w450, index=0) -> (element=w449:dbl)
            n348 = Index Array(array=w450, index=1) -> (element=w448:dbl)
            n349 = Index Array(array=w450, index=2) -> (element=w447:dbl)
            n350 = Index Array(array=w450, index=3) -> (element=w446:dbl)
            n351 = Number To Decimal String(number=w509) -> (decimal integer string=w508:string)  [unwired: 1 in]
            n352 = Number To Decimal String(number=w507) -> (decimal integer string=w506:string)  [unwired: 1 in]
            n353 = Number To Decimal String(number=w505) -> (decimal integer string=w504:string)  [unwired: 1 in]
            n354 = Number To Decimal String(number=w495) -> (decimal integer string=w492:string)  [unwired: 1 in]
            n355 = Number To Decimal String(number=w494) -> (decimal integer string=w491:string)  [unwired: 1 in]
            n356 = Number To Decimal String(number=w493) -> (decimal integer string=w490:string)  [unwired: 1 in]
            n357 = Number To Decimal String(number=w503) -> (decimal integer string=w502:string)  [unwired: 1 in]
            n358 = Number To Decimal String(number=w484) -> (decimal integer string=w480:string)  [unwired: 1 in]
            n359 = Number To Decimal String(number=w483) -> (decimal integer string=w479:string)  [unwired: 1 in]
            n360 = Number To Decimal String(number=w482) -> (decimal integer string=w478:string)  [unwired: 1 in]
            n361 = Number To Decimal String(number=w481) -> (decimal integer string=w477:string)  [unwired: 1 in]
            n362 = Number To Decimal String(number=w501) -> (decimal integer string=w500:string)  [unwired: 1 in]
            n363 = local read "Rolling Moment 2nd Polynomial Coefficients"() -> (w354:dbl[])
            n364 = local read "Rolling Moment 3rd Polynomial Coefficients"() -> (w343:dbl[])
            n365 = local read "P.M. 1st R-Squared"() -> (w436:dbl)
            n366 = local read "P.M. 1st Intercept"() -> (w437:dbl)
            n367 = local read "P.M. 2nd Residue"() -> (w434:dbl)
            n368 = local read "P.M. 3rd Residue"() -> (w435:dbl)
            n369 = local read "P.M. 1st Slope"() -> (w438:dbl)
            n370 = call "Build Axial"("Beginning Text"=w510, "axial_1st_1st_coef"=w508, "axial_1st_2nd_coef"=w506, "axial_1st_residue"=w504, "axial_2nd_1st_coef"=w492, "axial_2nd_2nd_coef"=w491, "axial_2nd_3rd_coef"=w490, "error in (no error)"=w476, "axial_2nd_residue"=w502, "axial_3rd_1st_coef"=w480, "axial_3rd_2nd_coef"=w479, "axial_3rd_3rd_coef"=w478, "axial_3rd_4th_coef"=w477, "axial_3rd_residue"=w500) -> ("Result"=w440:string, "error out"=w475:errorcluster)  [unwired: 12 in]
            n371 = Index Array(array=w428, index=0) -> (element=w422:dbl)
            n372 = Index Array(array=w428, index=1) -> (element=w421:dbl)
            n373 = Index Array(array=w428, index=2) -> (element=w420:dbl)
            n374 = Index Array(array=w427, index=0) -> (element=w426:dbl)
            n375 = Index Array(array=w427, index=1) -> (element=w425:dbl)
            n376 = Index Array(array=w427, index=2) -> (element=w424:dbl)
            n377 = Index Array(array=w427, index=3) -> (element=w423:dbl)
            n378 = Number To Decimal String(number=w474) -> (decimal integer string=w469:string)  [unwired: 1 in]
            n379 = Number To Decimal String(number=w473) -> (decimal integer string=w468:string)  [unwired: 1 in]
            n380 = Number To Decimal String(number=w472) -> (decimal integer string=w467:string)  [unwired: 1 in]
            n381 = Number To Decimal String(number=w454) -> (decimal integer string=w453:string)  [unwired: 1 in]
            n382 = Number To Decimal String(number=w455) -> (decimal integer string=w452:string)  [unwired: 1 in]
            n383 = Number To Decimal String(number=w456) -> (decimal integer string=w451:string)  [unwired: 1 in]
            n384 = Number To Decimal String(number=w471) -> (decimal integer string=w466:string)  [unwired: 1 in]
            n385 = Number To Decimal String(number=w449) -> (decimal integer string=w445:string)  [unwired: 1 in]
            n386 = Number To Decimal String(number=w448) -> (decimal integer string=w444:string)  [unwired: 1 in]
            n387 = Number To Decimal String(number=w447) -> (decimal integer string=w443:string)  [unwired: 1 in]
            n388 = Number To Decimal String(number=w446) -> (decimal integer string=w442:string)  [unwired: 1 in]
            n389 = Number To Decimal String(number=w470) -> (decimal integer string=w465:string)  [unwired: 1 in]
            n390 = local read "S.F. 1st R-Squared"() -> (w401:dbl)
            n391 = local read "S.F. 1st Intercept"() -> (w402:dbl)
            n392 = local read "S.F. 2nd Residue"() -> (w397:dbl)
            n393 = local read "S.F. 3rd Residue"() -> (w395:dbl)
            n394 = call "Build n"("Beginning Text"=w440, "n_1st_1st_coef"=w469, "n_1st_2nd_coef"=w468, "n_1st_residue"=w467, "n_2nd_1st_coef"=w453, "n_2nd_2nd_coef"=w452, "n_2nd_3rd_coef"=w451, "error in (no error)"=w475, "n_2nd_residue"=w466, "n_3rd_1st_coef"=w445, "n_3rd_2nd_coef"=w444, "n_3rd_3rd_coef"=w443, "n_3rd_4th_coef"=w442, "n_3rd_residue"=w465) -> ("Result"=w439:string, "error out"=w441:errorcluster)  [unwired: 12 in]
            n395 = local read "Rolling Moment 1st R-Squared"() -> (w365:dbl)
            n396 = Index Array(array=w387, index=1) -> (element=w392:dbl)
            n397 = Index Array(array=w387, index=2) -> (element=w391:dbl)
            n398 = Index Array(array=w387, index=0) -> (element=w393:dbl)
            n399 = Index Array(array=w378, index=0) -> (element=w386:dbl)
            n400 = Index Array(array=w378, index=1) -> (element=w385:dbl)
            n401 = Index Array(array=w378, index=2) -> (element=w384:dbl)
            n402 = Index Array(array=w378, index=3) -> (element=w383:dbl)
            n403 = Number To Decimal String(number=w438) -> (decimal integer string=w433:string)  [unwired: 1 in]
            n404 = Number To Decimal String(number=w437) -> (decimal integer string=w432:string)  [unwired: 1 in]
            n405 = Number To Decimal String(number=w436) -> (decimal integer string=w431:string)  [unwired: 1 in]
            n406 = Number To Decimal String(number=w422) -> (decimal integer string=w416:string)  [unwired: 1 in]
            n407 = Number To Decimal String(number=w421) -> (decimal integer string=w415:string)  [unwired: 1 in]
            n408 = Number To Decimal String(number=w420) -> (decimal integer string=w414:string)  [unwired: 1 in]
            n409 = Number To Decimal String(number=w434) -> (decimal integer string=w430:string)  [unwired: 1 in]
            n410 = Number To Decimal String(number=w426) -> (decimal integer string=w409:string)  [unwired: 1 in]
            n411 = Number To Decimal String(number=w425) -> (decimal integer string=w408:string)  [unwired: 1 in]
            n412 = Number To Decimal String(number=w424) -> (decimal integer string=w407:string)  [unwired: 1 in]
            n413 = Number To Decimal String(number=w423) -> (decimal integer string=w406:string)  [unwired: 1 in]
            n414 = Number To Decimal String(number=w435) -> (decimal integer string=w429:string)  [unwired: 1 in]
            n415 = local read "Rolling Moment 1st Intercept"() -> (w366:dbl)
            n416 = local read "Rolling Moment 2nd Residue"() -> (w364:dbl)
            n417 = local read "Rolling Moment 3rd Residue"() -> (w363:dbl)
            n418 = local read "Rolling Moment 1st Slope"() -> (w367:dbl)
            n419 = call "Build P.M."("Beginning Text"=w439, "pm_1st_1st_coef"=w433, "pm_1st_2nd_coef"=w432, "pm_1st_residue"=w431, "pm_2nd_1st_coef"=w416, "pm_2nd_2nd_coef"=w415, "pm_2nd_3rd_coef"=w414, "error in (no error)"=w441, "pm_2nd_residue"=w430, "pm_3rd_1st_coef"=w409, "pm_3rd_2nd_coef"=w408, "pm_3rd_3rd_coef"=w407, "pm_3rd_4th_coef"=w406, "pm_3rd_residue"=w429) -> ("Result"=w405:string, "error out"=w404:errorcluster)  [unwired: 12 in]
            n420 = Index Array(array=w354, index=0) -> (element=w353:dbl)
            n421 = Index Array(array=w354, index=1) -> (element=w352:dbl)
            n422 = Index Array(array=w354, index=2) -> (element=w351:dbl)
            n423 = Index Array(array=w343, index=0) -> (element=w342:dbl)
            n424 = Index Array(array=w343, index=1) -> (element=w341:dbl)
            n425 = Index Array(array=w343, index=2) -> (element=w340:dbl)
            n426 = Index Array(array=w343, index=3) -> (element=w339:dbl)
            n427 = Number To Decimal String(number=w402) -> (decimal integer string=w399:string)  [unwired: 1 in]
            n428 = Number To Decimal String(number=w401) -> (decimal integer string=w398:string)  [unwired: 1 in]
            n429 = Number To Decimal String(number=w392) -> (decimal integer string=w373:string)  [unwired: 1 in]
            n430 = Number To Decimal String(number=w391) -> (decimal integer string=w372:string)  [unwired: 1 in]
            n431 = Number To Decimal String(number=w393) -> (decimal integer string=w371:string)  [unwired: 1 in]
            n432 = Number To Decimal String(number=w397) -> (decimal integer string=w396:string)  [unwired: 1 in]
            n433 = Number To Decimal String(number=w386) -> (decimal integer string=w377:string)  [unwired: 1 in]
            n434 = Number To Decimal String(number=w385) -> (decimal integer string=w376:string)  [unwired: 1 in]
            n435 = Number To Decimal String(number=w384) -> (decimal integer string=w375:string)  [unwired: 1 in]
            n436 = Number To Decimal String(number=w383) -> (decimal integer string=w374:string)  [unwired: 1 in]
            n437 = Number To Decimal String(number=w395) -> (decimal integer string=w394:string)  [unwired: 1 in]
            n438 = call "Build S.F."("Beginning Text"=w405, "sf_1st_1st_coef"=w400, "sf_1st_2nd_coef"=w399, "sf_1st_residue"=w398, "sf_2nd_1st_coef"=w373, "sf_2nd_2nd_coef"=w372, "sf_2nd_3rd_coef"=w371, "error in (no error)"=w404, "sf_2nd_residue"=w396, "sf_3rd_1st_coef"=w377, "sf_3rd_2nd_coef"=w376, "sf_3rd_3rd_coef"=w375, "sf_3rd_4th_coef"=w374, "sf_3rd_residue"=w394) -> ("Result"=w370:string, "error out"=w334:errorcluster)  [unwired: 12 in]
            n439 = Number To Decimal String(number=w367) -> (decimal integer string=w362:string)  [unwired: 1 in]
            n440 = Number To Decimal String(number=w366) -> (decimal integer string=w361:string)  [unwired: 1 in]
            n441 = Number To Decimal String(number=w365) -> (decimal integer string=w360:string)  [unwired: 1 in]
            n442 = Number To Decimal String(number=w353) -> (decimal integer string=w350:string)  [unwired: 1 in]
            n443 = Number To Decimal String(number=w352) -> (decimal integer string=w349:string)  [unwired: 1 in]
            n444 = Number To Decimal String(number=w351) -> (decimal integer string=w348:string)  [unwired: 1 in]
            n445 = Number To Decimal String(number=w364) -> (decimal integer string=w359:string)  [unwired: 1 in]
            n446 = Number To Decimal String(number=w342) -> (decimal integer string=w338:string)  [unwired: 1 in]
            n447 = Number To Decimal String(number=w341) -> (decimal integer string=w337:string)  [unwired: 1 in]
            n448 = Number To Decimal String(number=w340) -> (decimal integer string=w336:string)  [unwired: 1 in]
            n449 = Number To Decimal String(number=w339) -> (decimal integer string=w335:string)  [unwired: 1 in]
            n450 = Number To Decimal String(number=w363) -> (decimal integer string=w358:string)  [unwired: 1 in]
            n451 = local read "Report Path"() -> (w369:path)
            n452 = call "Build Rolling"("Beginning Text"=w370, "rolling_1st_1st_coef"=w362, "rolling_1st_2nd_coef"=w361, "rolling_1st_residue"=w360, "rolling_2nd_1st_coef"=w350, "rolling_2nd_2nd_coef"=w349, "rolling_2nd_3rd_coef"=w348, "error in (no error)"=w334, "rolling_2nd_residue"=w359, "rolling_3rd_1st_coef"=w338, "rolling_3rd_2nd_coef"=w337, "rolling_3rd_3rd_coef"=w336, "rolling_3rd_4th_coef"=w335, "rolling_3rd_residue"=w358) -> ("Result"=w368:string, "error out"=w333:errorcluster)  [unwired: 12 in]
            n453 = Write to Text File(file (use dialog)=w369, text=w368, error in=w333) -> ()  [unwired: 1 in, 3 out]
          }
          frame #3 {
            # "Feature: Append Matrix to a file"
            n454 = local read "CSV Array"() -> (w549:dbl[][])
            n455 = local read "CSV Path"() -> (w552:path)
            n456 = local read "Report Path"() -> (w554:path)
            n457 = local read "Final Matrix"() -> (w555:T9)
            n458 = call-poly <vilib>:"Write Delimited Spreadsheet.vi"("file path (dialog if empty)"=w552, "format (%.3f)"="%.6f", "2D data"=w549, "append to file? (new file:F)"=FALSE, "delimiter (\\t)"="," ("delimiter (\\t)")) -> ()  [unwired: 9 in, 2 out]
            n459 = call-poly <vilib>:"Write Delimited Spreadsheet.vi"("file path (dialog if empty)"=w554, "format (%.3f)"="%.6f", "2D data"=w555, "append to file? (new file:F)"=TRUE) -> ()  [unwired: 10 in, 2 out]
          }
        }
      }
    }
  }
  n460 = while {
    stop <- FALSE stop-if-true
    n461 = event shown="[1] \"Add Weight\": Value Change" {
      selector: _ -> [_ _]
      dyn-events: _ -> [_ _]
      timeout: _ -> [_ _]
      event Timeout {
        n462 = event-data() -> ()  [unwired: 1 in, 3 out]
      }
      event "Add Weight": Value Change {
        # "Feature: Add Specified WEIGHT\nto the \"Weight\" array."
        n463 = event-data() -> ()  [unwired: 1 in, 6 out]
        n464 = local read "Weight"() -> (w558:dbl[])
        n465 = Insert Into Array(array=w558, new element="Weight to be added") -> (w557:dbl[])  [unwired: 1 in]
        n466 = local write "Weight"(w557) -> ()
      }
    }
  }
  n467 = while {
    stop <- FALSE stop-if-true
    # "Feature: Main Channel Selection"
    n468 = local read "Main Channel"() -> (w574:string)
    n469 = local read "Main Channel"() -> (w577:string)
    n470 = local read "Main Channel"() -> (w570:string)
    n471 = local read "Main Channel"() -> (w568:string)
    n472 = local read "Main Channel"() -> (w566:string)
    n473 = local read "Main Channel"() -> (w564:string)
    n474 = Equal?(x=w570, y="n") -> (x = y?=w571:bool)
    n475 = Equal?(x=w564, y="Rolling Moment") -> (x = y?=w565:bool)
    n476 = Equal?(x=w574, y="Axial Force") -> (x = y?=w573:bool)
    n477 = Equal?(x=w566, y="S.F.") -> (x = y?=w567:bool)
    n478 = Equal?(x=w577, y="Normal Force") -> (x = y?=w575:bool)
    n479 = Equal?(x=w568, y="P.M.") -> (x = y?=w569:bool)
    n480 = case shown="True" w575 {
      frame False {
      }
      frame True {
        n481 = local read "Voltage(Normal)"() -> (w584:dbl[])
        n482 = local write "Main Voltage"(w584) -> ()
      }
    }
    n483 = case shown="True" w573 {
      frame False {
      }
      frame True {
        n484 = local read "Voltage(Axial)"() -> (w583:dbl[])
        n485 = local write "Main Voltage"(w583) -> ()
      }
    }
    n486 = case shown="True" w571 {
      frame False {
      }
      frame True {
        n487 = local read "Voltage(n)"() -> (w582:dbl[])
        n488 = local write "Main Voltage"(w582) -> ()
      }
    }
    n489 = case shown="True" w569 {
      frame False {
      }
      frame True {
        n490 = local read "Voltage(P.M.)"() -> (w581:dbl[])
        n491 = local write "Main Voltage"(w581) -> ()
      }
    }
    n492 = case shown="True" w567 {
      frame False {
      }
      frame True {
        n493 = local read "Voltage(S.F.)"() -> (w580:dbl[])
        n494 = local write "Main Voltage"(w580) -> ()
      }
    }
    n495 = case shown="True" w565 {
      frame False {
      }
      frame True {
        n496 = local read "Voltage(R.M.)"() -> (w579:dbl[])
        n497 = local write "Main Voltage"(w579) -> ()
      }
    }
  }
  n498 = while {
    stop <- FALSE stop-if-true
    n499 = local read "Voltage(Normal)"() -> (w606:dbl[])
    n500 = local read "Voltage(Normal)"() -> (w591:dbl[])
    n501 = local read "Voltage(R.M.)"() -> (w599:dbl[])
    n502 = local read "Voltage(Axial)"() -> (w603:dbl[])
    n503 = local read "Voltage(P.M.)"() -> (w601:dbl[])
    n504 = local read "Voltage(Axial)"() -> (w590:dbl[])
    n505 = local read "Voltage(R.M.)"() -> (w586:dbl[])
    n506 = local read "Voltage(P.M.)"() -> (w588:dbl[])
    n507 = local read "Voltage(S.F.)"() -> (w600:dbl[])
    n508 = local read "Voltage(S.F.)"() -> (w587:dbl[])
    n509 = local read "Voltage(n)"() -> (w602:dbl[])
    n510 = local read "Voltage(n)"() -> (w589:dbl[])
    n511 = local read "Weight"() -> (w604:dbl[])
    n512 = local read "Weight"() -> (w592:dbl[])
    n513 = call-poly <vilib>:"Array To Matrix.vi"("Real 1D Array"=w604) -> ("Real Matrix (Column Vector)"=w605:T9)
    n514 = call-poly <vilib>:"Array To Matrix.vi"("Real 1D Array"=w606) -> ("Real Matrix (Column Vector)"=w607:T9)
    n515 = call-poly <vilib>:"Array To Matrix.vi"("Real 1D Array"=w603) -> ("Real Matrix (Column Vector)"=w598:T9)
    n516 = call-poly <vilib>:"Array To Matrix.vi"("Real 1D Array"=w602) -> ("Real Matrix (Column Vector)"=w597:T9)
    n517 = call-poly <vilib>:"Array To Matrix.vi"("Real 1D Array"=w601) -> ("Real Matrix (Column Vector)"=w596:T9)
    n518 = call-poly <vilib>:"Array To Matrix.vi"("Real 1D Array"=w600) -> ("Real Matrix (Column Vector)"=w595:T9)
    n519 = call-poly <vilib>:"Array To Matrix.vi"("Real 1D Array"=w599) -> ("Real Matrix (Column Vector)"=w594:T9)
    n520 = Build Array (concatenate)(w605, w607, w598, w597, w596, w595, w594) -> (w593:T9)
    n521 = Build Array(w592, w591, w590, w589, w588, w587, w586) -> (w585:dbl[][])
    n522 = local write "Final Matrix"(w593) -> ()
    n523 = local write "CSV Array"(w585) -> ()
  }
  n524 = while {
    stop <- FALSE stop-if-true
    # "Feature:\nMain Channel Selection and Indicator"
    "Current Main Channel Calibration" <- "Main Channel"
  }
  n525 = while {
    stop <- FALSE stop-if-true
    # "Feature: Clear ALL data from ALL arrays."
    n526 = event shown="[1] \"Clear Table\": Value Change" {
      selector: _ -> [_ _]
      dyn-events: _ -> [_ _]
      timeout: _ -> [_ _]
      event Timeout {
        n527 = event-data() -> ()  [unwired: 1 in, 3 out]
      }
      event "Clear Table": Value Change {
        n528 = event-data() -> ()  [unwired: 1 in, 6 out]
        n529 = local read "Voltage(Axial)"() -> (w630:dbl[])
        n530 = local read "Voltage(Normal)"() -> (w633:dbl[])
        n531 = local read "Main Voltage"() -> (w639:dbl[])
        n532 = local read "Voltage(n)"() -> (w627:dbl[])
        n533 = local read "Voltage(S.F.)"() -> (w619:dbl[])
        n534 = local read "Voltage(R.M.)"() -> (w615:dbl[])
        n535 = local read "Weight"() -> (w640:dbl[])
        n536 = local read "Voltage(P.M.)"() -> (w622:dbl[])
        n537 = Array Size(array=w640) -> (size(s)=w643:i32)
        n538 = Array Size(array=w630) -> (size(s)=w631:i32)
        n539 = Array Size(array=w627) -> (size(s)=w626:i32)
        n540 = Array Size(array=w633) -> (size(s)=w634:i32)
        n541 = Array Size(array=w639) -> (size(s)=w638:i32)
        n542 = Array Size(array=w619) -> (size(s)=w618:i32)
        n543 = Array Size(array=w622) -> (size(s)=w623:i32)
        n544 = Array Size(array=w615) -> (size(s)=w614:i32)
        n545 = Equal?(x=w643, y=0) -> (x = y?=w641:bool)
        n546 = Equal?(x=w631, y=0) -> (x = y?=w628:bool)
        n547 = Equal?(x=w626, y=0) -> (x = y?=w624:bool)
        n548 = Equal?(x=w618, y=0) -> (x = y?=w616:bool)
        n549 = Equal?(x=w614, y=0) -> (x = y?=w613:bool)
        n550 = Equal?(x=w623, y=0) -> (x = y?=w620:bool)
        n551 = Equal?(x=w634, y=0) -> (x = y?=w635:bool)
        n552 = Equal?(x=w638, y=0) -> (x = y?=w636:bool)
        n553 = case shown="False" w628 {
          frame False {
            n554 = local read "Voltage(Axial)"() -> (w665:dbl[])
            n555 = Array Size(array=w665) -> (size(s)=w664:i32)
            n556 = for {
              N: w664 -> [_]
              n557 = local read "Voltage(Axial)"() -> (w668:dbl[])
              n558 = Delete From Array(array=w668, index=0) -> (array with subset deleted=w666:dbl[])  [unwired: 1 in, 1 out]
              n559 = local write "Voltage(Axial)"(w666) -> ()
            }
          }
          frame True {
          }
        }
        n560 = case shown="False" w624 {
          frame False {
            n561 = local read "Voltage(n)"() -> (w660:dbl[])
            n562 = Array Size(array=w660) -> (size(s)=w659:i32)
            n563 = for {
              N: w659 -> [_]
              n564 = local read "Voltage(n)"() -> (w663:dbl[])
              n565 = Delete From Array(array=w663, index=0) -> (array with subset deleted=w661:dbl[])  [unwired: 1 in, 1 out]
              n566 = local write "Voltage(n)"(w661) -> ()
            }
          }
          frame True {
          }
        }
        n567 = case shown="False" w620 {
          frame False {
            n568 = local read "Voltage(P.M.)"() -> (w655:dbl[])
            n569 = Array Size(array=w655) -> (size(s)=w654:i32)
            n570 = for {
              N: w654 -> [_]
              n571 = local read "Voltage(P.M.)"() -> (w658:dbl[])
              n572 = Delete From Array(array=w658, index=0) -> (array with subset deleted=w656:dbl[])  [unwired: 1 in, 1 out]
              n573 = local write "Voltage(P.M.)"(w656) -> ()
            }
          }
          frame True {
          }
        }
        n574 = case shown="False" w616 {
          frame False {
            n575 = local read "Voltage(S.F.)"() -> (w650:dbl[])
            n576 = Array Size(array=w650) -> (size(s)=w649:i32)
            n577 = for {
              N: w649 -> [_]
              n578 = local read "Voltage(S.F.)"() -> (w653:dbl[])
              n579 = Delete From Array(array=w653, index=0) -> (array with subset deleted=w652:dbl[])  [unwired: 1 in, 1 out]
              n580 = local write "Voltage(S.F.)"(w652) -> ()
            }
          }
          frame True {
          }
        }
        n581 = case shown="False" w613 {
          frame False {
            n582 = local read "Voltage(R.M.)"() -> (w644:dbl[])
            n583 = Array Size(array=w644) -> (size(s)=w645:i32)
            n584 = for {
              N: w645 -> [_]
              n585 = local read "Voltage(R.M.)"() -> (w648:dbl[])
              n586 = Delete From Array(array=w648, index=0) -> (array with subset deleted=w646:dbl[])  [unwired: 1 in, 1 out]
              n587 = local write "Voltage(R.M.)"(w646) -> ()
            }
          }
          frame True {
          }
        }
        n588 = case shown="False" w635 {
          frame False {
            n589 = local read "Voltage(Normal)"() -> (w670:dbl[])
            n590 = Array Size(array=w670) -> (size(s)=w669:i32)
            n591 = for {
              N: w669 -> [_]
              n592 = local read "Voltage(Normal)"() -> (w673:dbl[])
              n593 = Delete From Array(array=w673, index=0) -> (array with subset deleted=w672:dbl[])  [unwired: 1 in, 1 out]
              n594 = local write "Voltage(Normal)"(w672) -> ()
            }
          }
          frame True {
          }
        }
        n595 = case shown="False" w641 {
          frame False {
            n596 = local read "Weight"() -> (w680:dbl[])
            n597 = Array Size(array=w680) -> (size(s)=w679:i32)
            n598 = for {
              N: w679 -> [_]
              n599 = local read "Weight"() -> (w682:dbl[])
              n600 = Delete From Array(array=w682, index=0) -> (array with subset deleted=w681:dbl[])  [unwired: 1 in, 1 out]
              n601 = local write "Weight"(w681) -> ()
            }
          }
          frame True {
          }
        }
        n602 = case shown="False" w636 {
          frame False {
            n603 = local read "Main Voltage"() -> (w675:dbl[])
            n604 = Array Size(array=w675) -> (size(s)=w674:i32)
            n605 = for {
              N: w674 -> [_]
              n606 = local read "Main Voltage"() -> (w677:dbl[])
              n607 = Delete From Array(array=w677, index=0) -> (array with subset deleted=w678:dbl[])  [unwired: 1 in, 1 out]
              n608 = local write "Main Voltage"(w678) -> ()
            }
          }
          frame True {
          }
        }
      }
    }
  }
  "Matrix Path Indicator" <- "Report Path"
